vi "CMN_ConfigVals.vi"(8 "error in (no error)":errorcluster, 9 "Action":enum16{"Read from File", "Write to File"}(ring), 10 "ConfigVariables":string[][](table)=[["MODULE", "Name", "FLT_Glbs.vi", "FLT_FilterModule", "NONE", "STR"], ["FILTERS", "Path", "FLT_Glbs.vi", "FLT_FilterConfig", "NONE", "PATH"]], 11 "configuration file path":path=path "/home/ArcVIEW/ConfigFiles/ctiocameragui.cfg") -> (0 "error out":errorcluster)   [LabVIEW 2016]
uses:
  <vilib>/Utility/config.llb/Read Key (String).vi
  <vilib>/Utility/config.llb/Write Key (String).vi
  <vilib>/Utility/config.llb/NI_LVConfig.lvlib
panel:
  # "default value"
  # "Ctrl type"
  # "Ctrl name"
  # "Seccion"
  # "Vi name"
  # "Keyword"
  # "if read is TRUE, then maps the specified keyword, which\nis on the specified seccion, to the specified control in the specified\nvi. If the keyword/seccion pairs are not found, then puts on the control the\n default value specified.\nif read is FALSE, then writes the value of the control to the specified \nkey on the specified seccion."
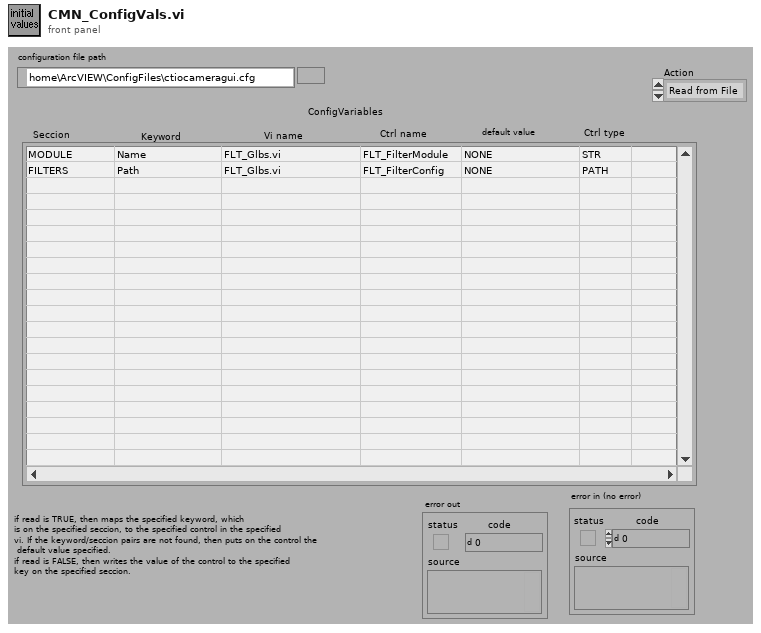
[diagram p1: front panel]
types:
  T1 = typedef "NI_LVConfig.lvlib/Config Data RefNum.ctl" = refnum<k1>
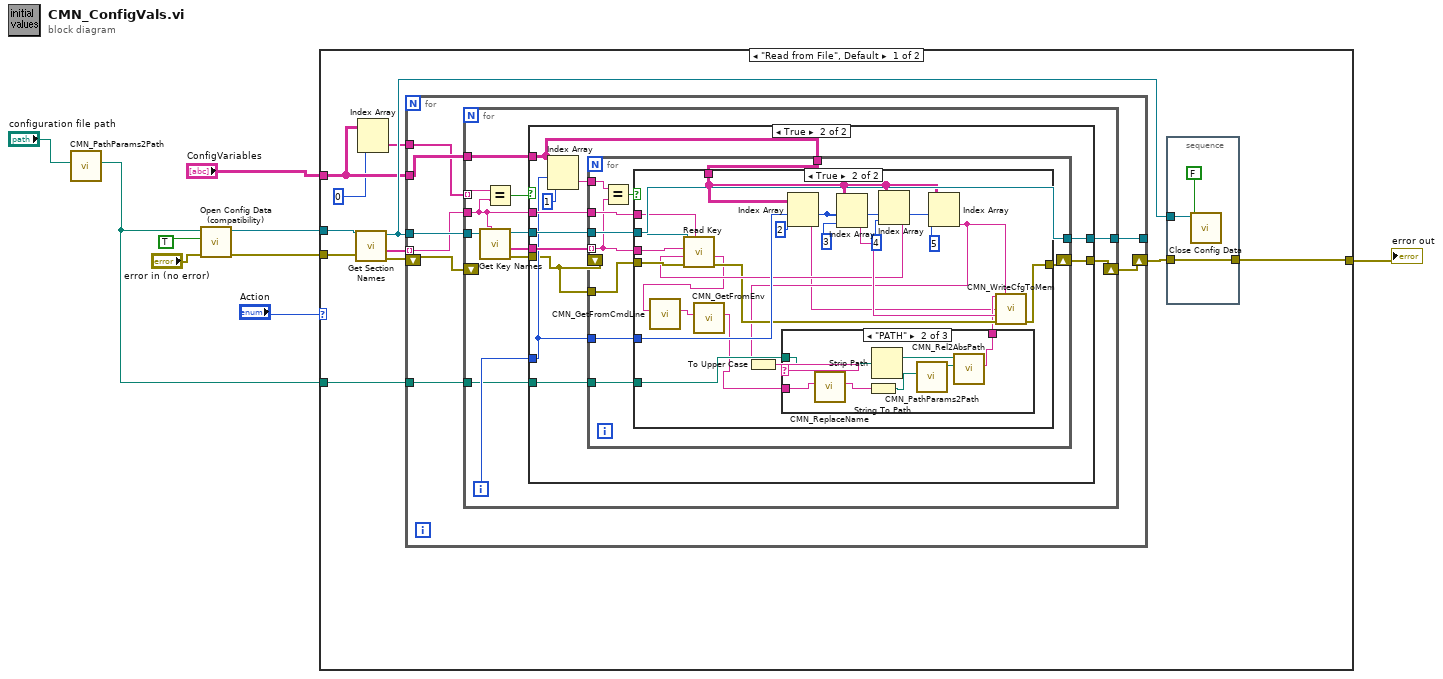
[diagram p0: block diagram]
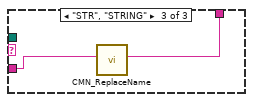
[diagram p5: hidden frame]
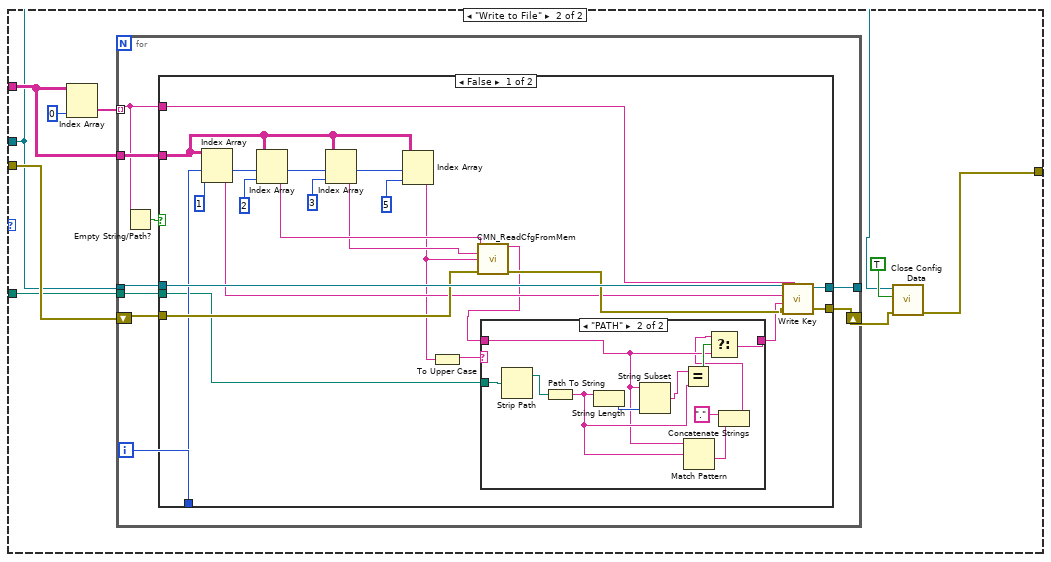
[diagram p6: hidden frame]
diagram:
  n1 = call "CMN_PathParams2Path.vi"("Path In"="configuration file path") -> ("Path out"=w1:path)  [unwired: 2 in, 8 out]
  n2 = call <vilib>:"Open Config Data (compatibility).vi"("error in (no error)"="error in (no error)", "create file if necessary (T)"=TRUE ("create file if necessary? (T)"), "configuration file path"=w1) -> ("error out"=w8:errorcluster, "refnum"=w7:T1)  [unwired: 6 in, 1 out]
  n3 = case shown="\"Read from File\", Default" "Action" {
    tunnel: w8 -> [w20 w105]
    tunnel: w7 -> [w19 w100]
    tunnel: [w14 w103] -> w6
    tunnel: "ConfigVariables" -> [w12 w106]
    tunnel: w1 -> [w16 w101]
    frame "Read from File", Default {
      n4 = call <vilib>:"Get Section Names.vi"("error in (no error)"=w20, "refnum"=w19) -> ("error out"=w18:errorcluster, "section names"=w17:string[], "refnum out"=w13:T1)  [unwired: 7 out]
      n5 = Index Array(array=w12, index (col)=0 ("Disabled Index (col)")) -> (element=w10:string[])  [unwired: 1 in]
      n6 = for {
        tunnel: w13 -> [w31]
        tunnel: [w30] -> _
        shift-right: [w26] -> w15
        shift-left: w18 -> [w27]
        tunnel: w17 -> [w29] mode=indexing
        tunnel: w12 -> [w28]
        tunnel: w16 -> [w25]
        tunnel: w10 -> [w24]
        n7 = for {
          tunnel: w31 -> [w43]
          tunnel: [w42] -> w30
          tunnel: w29 -> [w37]
          tunnel: w24 -> [w38] mode=indexing
          tunnel: w28 -> [w35]
          shift-right: [w33] -> w26
          shift-left: w27 -> [_]
          tunnel: w25 -> [w32]
          i -> [w34]
          n8 = call <vilib>:"Get Key Names.vi"("section"=w37, "refnum"=w43) -> ("error out"=w39:errorcluster, "key names"=w41:string[], "refnum out"=w40:T1)  [unwired: 1 in, 6 out]
          n9 = Equal?(x=w38, y=w37) -> (x = y?=w36:bool)
          n10 = case shown="True" w36 {
            tunnel: [w44 w56] -> w42
            tunnel: [w45 w55] -> w33
            tunnel: w41 -> [_ w54]
            tunnel: w40 -> [w44 w53]
            tunnel: w39 -> [w45 w46]
            tunnel: w37 -> [_ w52]
            tunnel: w35 -> [_ w49]
            tunnel: w34 -> [_ w48]
            tunnel: w32 -> [_ w47]
            frame False {
            }
            frame True {
              n11 = Index Array(array=w49, index (row)=w48, index (col)=1) -> (element=w50:string)
              n12 = for {
                tunnel: w54 -> [w63] mode=indexing
                tunnel: w53 -> [w65]
                shift-right: [w66] -> w55
                shift-left: w46 -> [_]
                tunnel: [w65] -> w56
                tunnel: w52 -> [w64]
                tunnel: w50 -> [w62]
                tunnel: w49 -> [w60]
                tunnel: w48 -> [w59]
                tunnel: w47 -> [w58]
                tunnel: w46 -> [w57]
                n13 = Equal?(x=w62, y=w63) -> (x = y?=w61:bool)
                n14 = case shown="True" w61 {
                  tunnel: w63 -> [_ w89]
                  tunnel: w57 -> [w67 w88]
                  tunnel: [w67 w76] -> w66
                  tunnel: w65 -> [_ w87]
                  tunnel: w64 -> [_ w86]
                  tunnel: w60 -> [_ w82]
                  tunnel: w59 -> [_ w81]
                  tunnel: w58 -> [_ w75]
                  frame False {
                  }
                  frame True {
                    n15 = Index Array(array=w82, index (row)=w81, index (col)=2 ("Disabled Index (col)")) -> (element=w70:string)
                    n16 = Index Array(array=w82, index (row)=w81, index (col)=3 ("Disabled Index (col)")) -> (element=w79:string)
                    n17 = Index Array(array=w82, index (row)=w81, index (col)=4 ("Disabled Index (col)")) -> (element=w78:string)
                    n18 = call-poly <vilib>:"Read Key.vi"("section"=w86, "error in (no error)"=w88, "default value"=w78, "key"=w89, "refnum"=w87) -> ("error out"=w77:errorcluster, "value"=w71:string)  [unwired: 1 in, 4 out]
                    n19 = call "CMN_GetFromCmdLine.vi"("str in"=w71) -> ("str out"=w69:string)  [unwired: 10 out]
                    n20 = call "CMN_GetFromEnv.vi"("str in"=w69) -> ("str out"=w68:string)  [unwired: 10 out]
                    n21 = Index Array(array=w82, index (row)=w81, index (col)=5 ("Disabled Index (col)")) -> (element=w74:string)
                    n22 = To Upper Case(1:w74) -> (0:w73:string)
                    n23 = case shown="\"PATH\"" w73 {
                      tunnel: w75 -> [_ w93 _]
                      tunnel: w68 -> [w90 w92 w99]
                      tunnel: [w90 w97 w98] -> w72
                      frame Default {
                      }
                      frame "PATH" {
                        n24 = call "CMN_ReplaceName.vi"("name in"=w92) -> ("name out"=w91:string)  [unwired: 1 in, 9 out]
                        n25 = String To Path(string=w91) -> (path=w95:path)
                        n26 = Strip Path(path=w93) -> (stripped path=w96:path)  [unwired: 1 out]
                        n27 = call "CMN_PathParams2Path.vi"("Path In"=w95) -> ("Path out"=w94:path)  [unwired: 2 in, 8 out]
                        n28 = call "CMN_Rel2AbsPath.vi"("test path"=w94, "absolute path"=w96) -> ("output path (str)"=w97:string)  [unwired: 1 in, 8 out]
                      }
                      frame "STR", "STRING" {
                        n29 = call "CMN_ReplaceName.vi"("name in"=w99) -> ("name out"=w98:string)  [unwired: 1 in, 9 out]
                      }
                    }
                    n30 = call "CMN_WriteCfgToMem.vi"("Value"=w72, "Ctrl type"=w74, "Vi name"=w70, "Ctrl name"=w79, "error in"=w77) -> ("error out"=w76:errorcluster)  [unwired: 10 out]
                  }
                }
              }
            }
          }
        }
      }
      n31 = stacked-sequence {
        tunnel: w15 -> [w22]
        tunnel: [w22] -> w14
        tunnel: w13 -> [w21]
        frame #0 {
          n32 = call <vilib>:"Close Config Data.vi"("write file if changed (T)"=FALSE ("write configuration file? (T)"), "refnum"=w21) -> ()  [unwired: 1 in, 9 out]
        }
      }
    }
    frame "Write to File" {
      n33 = Index Array(array=w106, index (col)=0 ("Disabled Index (col)")) -> (element=w107:string[])  [unwired: 1 in]
      n34 = for {
        tunnel: w107 -> [w110] mode=indexing
        tunnel: w106 -> [w117]
        tunnel: w100 -> [w116]
        shift-right: [w115] -> w104
        shift-left: w105 -> [w114]
        tunnel: [w112] -> _
        tunnel: w101 -> [w109]
        i -> [w113]
        n35 = Empty String/Path?(string/path=w110) -> (empty?=w111:bool)
        n36 = case shown="False" w111 {
          tunnel: w117 -> [w137 _]
          tunnel: w116 -> [w134 w151]
          tunnel: [w133 w150] -> w115
          tunnel: w114 -> [w132 w150]
          tunnel: w110 -> [w130 _]
          tunnel: w113 -> [w128 _]
          tunnel: [w123 w151] -> w112
          tunnel: w109 -> [w118 _]
          frame False {
            n37 = Index Array(array=w137, index (row)=w128, index (col)=1 ("Disabled Index (col)")) -> (element=w129:string)
            n38 = Index Array(array=w137, index (row)=w128, index (col)=2 ("Disabled Index (row)")) -> (element=w136:string)
            n39 = Index Array(array=w137, index (row)=w128, index (col)=3 ("Disabled Index (row)")) -> (element=w135:string)
            n40 = Index Array(array=w137, index (row)=w128, index (col)=5 ("Disabled Index (row)")) -> (element=w121:string)
            n41 = To Upper Case(1:w121) -> (0:w122:string)
            n42 = call "CMN_ReadCfgFromMem.vi"("Vi name"=w136, "Control Name"=w135, "Type"=w121, "error in"=w132) -> ("Value"=w120:string, "error out"=w131:errorcluster)  [unwired: 10 out]
            n43 = case shown="\"PATH\"" w122 {
              tunnel: w120 -> [w138 w142]
              tunnel: [w138 w148] -> w119
              tunnel: w118 -> [_ w149]
              frame Default {
              }
              frame "PATH" {
                n44 = Strip Path(path=w149) -> (stripped path=w147:path)  [unwired: 1 out]
                n45 = Path To String(path=w147) -> (string=w143:string)
                n46 = String Length(string=w143) -> (length=w145:i32)
                n47 = String Subset(string=w142, length (rest)=w145) -> (substring=w144:string)  [unwired: 1 out]
                n48 = Equal?(x=w144, y=w143) -> (x = y?=w146:bool)
                n49 = Match Pattern(string=w142, regular expression=w143) -> (after substring=w141:string)  [unwired: 4 out]
                n50 = Concatenate Strings("." ("string"), w141) -> (w139:string)
                n51 = Select(t=w139, s=w146, f=w142) -> (s? t:f=w148:string)
              }
            }
            n52 = call-poly <vilib>:"Write Key.vi"("section"=w130, "error in (no error)"=w131, "value"=w119, "key"=w129, "refnum"=w134) -> ("error out"=w133:errorcluster, "refnum out"=w123:T1)  [unwired: 1 in, 4 out]
          }
          frame True {
          }
        }
      }
      n53 = call <vilib>:"Close Config Data.vi"("error in (no error)"=w104, "write file if changed (T)"=TRUE ("write configuration file? (F)"), "refnum"=w100) -> ("error out"=w103:errorcluster)  [unwired: 8 out]
    }
  }
  "error out" <- w6
